vi "deinitialize.vi"(0 "HGF_IMAQDevice":refnum<class "HGF_IMAQDevice.lvclass">, 5 "error in (no error)":errorcluster) -> (19 "error out":errorcluster)   [LabVIEW 2014, in "HGF_IMAQ.lvlib" / "HGF_IMAQDevice.lvclass"]
doc: "This is a dynamic dispatch VI. It can be overwritten by childclasses to release allocated recources."
uses:
  HGF_IMAQDevice.lvclass
  HGF_DeviceBaseClasses/HGF_DeviceBase/HGF_DeviceBase.lvclass
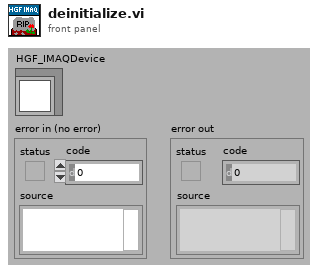
[diagram p1: front panel]
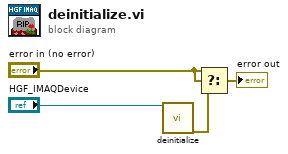
[diagram p0: block diagram]
diagram:
  n1 = call-parent "deinitialize.vi"("HGF_DeviceBase"="HGF_IMAQDevice") -> ("error out"=w3:errorcluster)  [unwired: 1 in, 17 out]
  n2 = Select(t="error in (no error)", s="error in (no error)", f=w3) -> (s? t:f=→"error out":errorcluster)
